vi "Shutdown State Machine Loop.vi"() -> ()   [LabVIEW 2014]
uses:
  Shutdown State Machine.lvsc/State.ctl
  Shutdown State Machine.lvsc/Inputs.ctl
  Shutdown State Machine.lvsc/StatechartState.ctl
  Shutdown State Machine.lvsc/CompanionDiagram.vi/7/SC Main.vi
  Shutdown State Machine.lvsc/CompanionDiagram.vi/7/Upd State.vi
  Shutdown State Machine.lvsc/CompanionDiagram.vi/7/Trans Graph0.vi
  Shutdown State Machine.lvsc/CompanionDiagram.vi/7/EnterGraphCore.vi
  <vilib>/FPGAPlugInAG/sbRIO-9626/niLvFpga_Open_sbRIO-9626.vi
  Global Data.vi
  <vilib>/Utility/error.llb/Error Cluster From Error Code.vi
  <vilib>/rvi/errors/niLvFpgaAdjustHostInterfaceError.vi
  Shutdown State Machine.lvsc/CompanionDiagram.vi
  <vilib>/FPGAPlugInAG/sbRIO-9626/niLvFpga_Close_sbRIO-9626.vi
  <vilib>/rvi/interface/common/dynamic/niFpgaDynamicAddResources.vi
  <vilib>/FPGAPlugInAG/Dynamic/niLvFpga_Close_Dynamic.vi
  <vilib>/rvi/interface/nirviOpenFPGA/nirviOpenFPGA.xnode
  FPGA Bitfiles/FormulaElectric2_FPGATarget_FPGA_8a5J0mMac2U.lvbitx
  Shutdown State Machine.lvsc/Trigger.ctl
  <vilib>/rvi/interface/nirviReadWriteControl/nirviReadWriteControl.xnode
  <vilib>/Statechart/Infrastructure/RTStatechart/RunTime SCN.xnode
  Shutdown State Machine.lvsc/Outputs.ctl
  AIR Status.ctl
  Shutdown State Machine.lvsc
  <vilib>/rvi/interface/nirviCloseFPGA/nirviCloseFPGA.xnode
  FPGA/Sensor Library/FPGA.vi
  NiFpgaLv.dll
  <vilib>/rvi/interface/Simulation/niFpgaSimulationCallBeginRW.vi
panel:
  out "Shutdown State":T1=enum."TSMS Off"
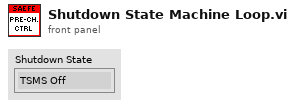
[diagram p1: front panel]
types:
  T1 = typedef "Shutdown State Machine.lvsc/State.ctl" = enum16{"NI.SC.Initial", "NI.SC.History", "NI.SC.ShallowHistory", "NI.SC.Terminal", "Coolant Pump Started/AIR's On", "AIRs On", "Precharge", "TSMS Off"}
  T2 = typedef "Shutdown State Machine.lvsc/Inputs.ctl" = cluster{"TSMS Status In":bool, "Precharge Time":u32}
  T3 = typedef "Shutdown State Machine.lvsc/Outputs.ctl" = cluster{"Positive AIR Enable":bool, "AIR Status":T4, "Coolant Pump":bool, "Precharge Failed":bool}
  T4 = typedef "AIR Status.ctl" = enum16{"Off", "Precharge", "On"}
  T5 = typedef "Shutdown State Machine.lvsc/StatechartState.ctl" = T1[]
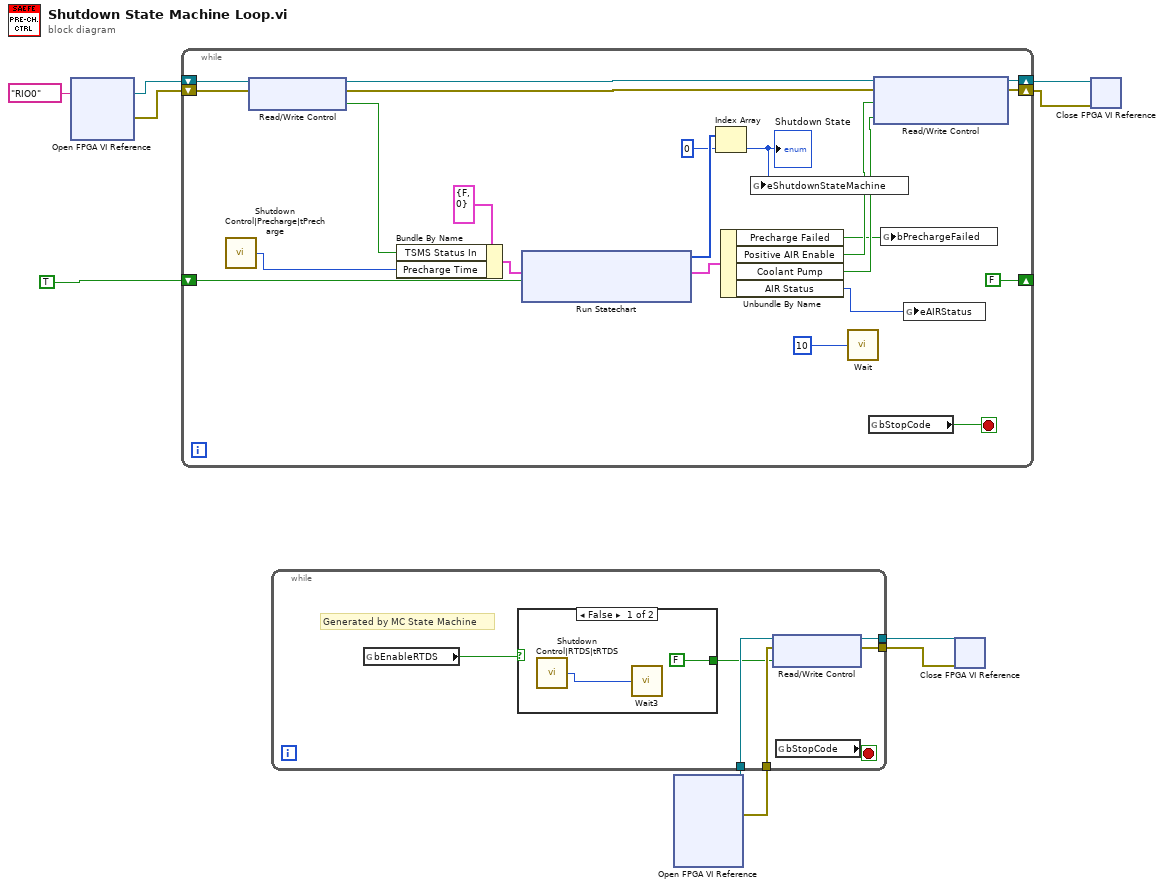
[diagram p0: block diagram]
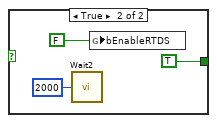
[diagram p2: hidden frame]
diagram:
  n1 = xnode "Open FPGA VI Reference"("resource name"=tag "RIO0") -> ("FPGA VI Reference Out"=w10:refnum<k20>, "error out"=w9:errorcluster)  [unwired: 1 in]
  n2 = while {
    shift-right: [FALSE] -> _
    shift-left: TRUE -> [w27]
    shift-right: [w14] -> w3
    shift-left: w10 -> [w32]
    shift-right: [w13] -> w2
    shift-left: w9 -> [w31]
    stop <- w17 stop-if-true
    n3 = call "Shutdown Control|Precharge|tPrecharge"() -> ("Value"=w11:u32)
    n4 = xnode "Read/Write Control"("FPGA VI Reference In"=w32, "error in"=w31) -> ("FPGA VI Reference Out"=w29:refnum<k20>, "error out"=w28:errorcluster, "bTSMSInStatus"=w23:bool)
    n5 = Bundle By Name(cluster=T2 {"TSMS Status In"=FALSE, "Precharge Time"=0} ("Inputs"), "TSMS Status In"=w23, "Precharge Time"=w11) -> (w24:T2)
    n6 = xnode "Run Statechart"("Init?"=w27, "Inputs"=w24) -> ("Outputs"=w22:T3, "Active States"=w21:T5)  [unwired: 1 in, 1 out]
    n7 = Index Array(array=w21, index=0) -> (element=w19:T1)
    "Shutdown State" <- w19
    n8 = Unbundle By Name(w22) -> ("Precharge Failed"=w12:bool, "Positive AIR Enable"=w16:bool, "Coolant Pump"=w15:bool, "AIR Status"=w18:T4)
    n9 = global write "Global Data.vi" "eShutdownStateMachine"(w19) -> ()
    n10 = call "Wait"("Count(mSec)"=u32 10) -> ()  [unwired: 1 out]
    n11 = global read "Global Data.vi" "bStopCode"() -> (w17:bool)
    n12 = xnode "Read/Write Control"("FPGA VI Reference In"=w29, "error in"=w28, "bPosAIREnable"=w16, "bCoolantPumpEnable"=w15) -> ("FPGA VI Reference Out"=w14:refnum<k20>, "error out"=w13:errorcluster)
    n13 = global write "Global Data.vi" "bPrechargeFailed"(w12) -> ()
    n14 = global write "Global Data.vi" "eAIRStatus"(w18) -> ()
  }
  n15 = xnode "Open FPGA VI Reference"() -> ("FPGA VI Reference Out"=w6:refnum<k20>, "error out"=w5:errorcluster)  [unwired: 2 in]
  n16 = while {
    tunnel: [w74] -> w8
    tunnel: [w73] -> w7
    tunnel: w6 -> [w72]
    tunnel: w5 -> [w71]
    stop <- w69 stop-if-true
    # "Generated by MC State Machine"
    n17 = global read "Global Data.vi" "bEnableRTDS"() -> (w75:bool)
    n18 = case shown="False" w75 {
      tunnel: [FALSE TRUE] -> w70
      frame False {
        n19 = call "Shutdown Control|RTDS|tRTDS"() -> ("Value"=w76:u32)
        n20 = call "Wait3"("Count(mSec)"=w76) -> ()  [unwired: 1 out]
      }
      frame True {
        n21 = call "Wait2"("Count(mSec)"=u32 2000) -> ()  [unwired: 1 out]
        n22 = global write "Global Data.vi" "bEnableRTDS"(FALSE ("Make Sound?")) -> ()
      }
    }
    n23 = xnode "Read/Write Control"("FPGA VI Reference In"=w72, "error in"=w71, "bRTDSEnable"=w70) -> ("FPGA VI Reference Out"=w74:refnum<k20>, "error out"=w73:errorcluster)
    n24 = global read "Global Data.vi" "bStopCode"() -> (w69:bool)
  }
  n25 = xnode "Close FPGA VI Reference"("FPGA VI Reference In"=w8, "error in"=w7) -> ()  [unwired: 1 out]
  n26 = xnode "Close FPGA VI Reference"("FPGA VI Reference In"=w3, "error in"=w2) -> ()  [unwired: 1 out]
